vi "Status.vi"(8 "error in (no error)":errorcluster, 11 "App ID in":u16) -> (0 "error out":errorcluster, 1 "Connected?":bool[](array[boolean]), 2 "Server Ports":u16[](array[numeric]), 3 "App ID out":u16, 4 "Server Port Types":enum8{"CMD", "TLM", "BOTH"}[](array[ring]), 5 "Client IP:Ports":string[](array[string]), 7 "Client Conns":refnum<k5>[](array[refnum]))   [LabVIEW 2018, in "TCPServer.lvlib"]
uses:
  TCPServer.lvlib
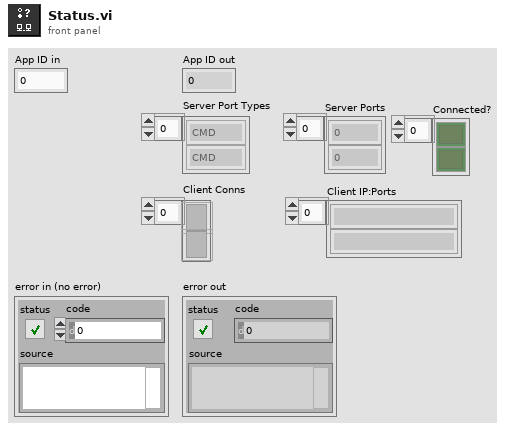
[diagram p1: front panel]
types:
  T1 = typedef "TCPServer.lvlib/App.ctl" = cluster{"Stack":refnum<queue>, "Cmd":cluster{"Conn":refnum<data-value>, "Daemon":refnum<vi>, "Counter":refnum<data-value>}, "Tlm":cluster{"Conn":refnum<data-value>, "Daemon":refnum<vi>, "Counter":refnum<data-value>}}
  T2 = typedef "TCPServer.lvlib/Connection.ctl" = cluster{"Tcp":refnum<k5>, "Server Port":u16, "Server Port Type":enum8{"CMD", "TLM", "BOTH"}, "Client IP":string, "Client Port":u16}
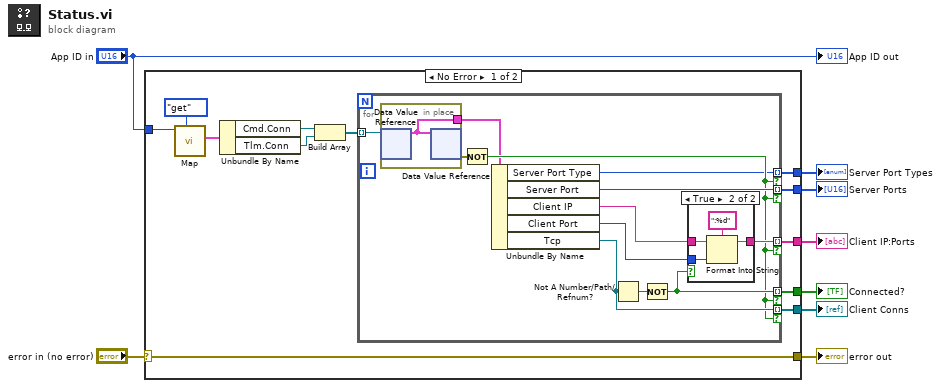
[diagram p0: block diagram]
diagram:
  n1 = case shown="No Error" "error in (no error)" {
    selector: "error in (no error)" -> [w15 w38]
    tunnel: [w19 _] -> w1
    tunnel: [w18 _] -> w8
    tunnel: [w17 _] -> w7
    tunnel: [w16 _] -> w6
    tunnel: [w15 w38] -> w5
    tunnel: "App ID in" -> [w14 _]
    tunnel: [w9 _] -> w2
    frame No Error {
      n2 = call "Map.vi"("Action"=enum8{"noop", "get", "set", "pop"}."get", "App ID in"=w14) -> ("App out"=w12:T1)  [unwired: 7 in, 2 out]
      n3 = Unbundle By Name(w12) -> ("Cmd.Conn"=w20:refnum<data-value>, "Tlm.Conn"=w10:refnum<data-value>)
      n4 = Build Array(w20, w10) -> (w11:refnum<data-value>[])
      n5 = for {
        tunnel: w11 -> [w32] mode=indexing
        tunnel: [w21] -> w19 mode=indexing if=w23
        tunnel: [w31] -> w16 mode=indexing if=w23
        tunnel: [w26] -> w17 mode=indexing if=w23
        tunnel: [w25] -> w18 mode=indexing if=w23
        tunnel: [w24] -> w9 mode=indexing if=w23
        n6 = in-place {
          in-place-border: [w33] -> w22
          n7 = in-place-dvr #1(w32) -> (w33:T2)  [unwired: 1 out]
          n8 = in-place-dvr #1(w33) -> (w29:errorcluster)  [unwired: 1 out]
        }
        n9 = Not(x=w29) -> (.not. x?=w23:bool)
        n10 = Unbundle By Name(w22) -> ("Server Port Type"=w21:enum8{"CMD", "TLM", "BOTH"}, "Server Port"=w31:u16, "Client IP"=w27:string, "Client Port"=w28:u16, "Tcp"=w24:refnum<k5>)
        n11 = Not A Number/Path/Refnum?(number/path/refnum=w24) -> (NaN/Path/Refnum?=w30:bool)
        n12 = Not(x=w30) -> (.not. x?=w25:bool)
        n13 = case shown="True" w25 {
          tunnel: w28 -> [_ w37]
          tunnel: w27 -> [_ w35]
          tunnel: [_ w34] -> w26
          frame False {
          }
          frame True {
            n14 = Format Into String(format string=":%d", initial string=w35, w37) -> (resulting string=w34:string)  [unwired: 1 in, 1 out]
          }
        }
      }
    }
    frame Error {
    }
  }
  "error out" <- w5
  "Connected?" <- w8
  "Client IP:Ports" <- w7
  "Server Ports" <- w6
  "Server Port Types" <- w1
  "Client Conns" <- w2
  "App ID out" <- "App ID in"
